vi "constant--tour_in_progress.vi"() -> (0 "blank_tour_in_progress":T1)   [LabVIEW 2020, in "core.lvlib" / "core_data.lvlib"]
uses:
  core_data.lvlib
  tour_in_progress.ctl
  chessboard_index.ctl
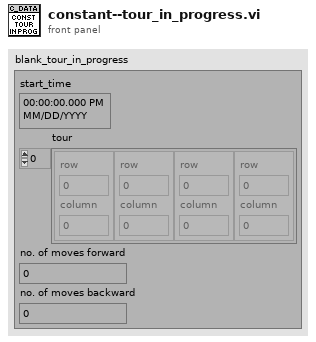
[diagram p1: front panel]
types:
  T1 = typedef "core.lvlib/core_data.lvlib/tour_in_progress.ctl" = cluster{"start_time":timestamp, "tour":T2[], "no. of moves forward":u64, "no. of moves backward":u64}
  T2 = typedef "core.lvlib/core_data.lvlib/chessboard_index.ctl" = cluster{"row":u8, "column":u8}
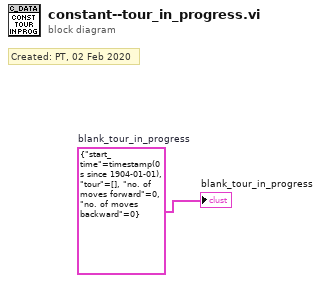
[diagram p0: block diagram]
diagram:
  w1 = T1 {"start_time"=timestamp(0 s since 1904-01-01), "tour"=[], "no. of moves forward"=0, "no. of moves backward"=0}  # blank_tour_in_progress
  # "Created: PT, 02 Feb 2020"
  "blank_tour_in_progress" <- w1
